vi "test global access to variables.vi"(1 "command":enum16{"read", "write"}(ring), 2 "Current Control settings":T1 {"Pump speed" format="%.2f"}) -> (0 "Current Control settings out":T1 {"Pump speed" format="%.2f"})   [LabVIEW 2010]
uses:
  Stamp Controls.ctl
  switches.ctl
panel:
  # "rpm"
  # "rpm"
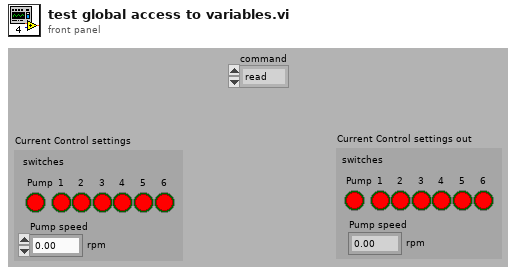
[diagram p1: front panel]
types:
  T1 = typedef "Stamp Controls.ctl" = cluster{"Pump speed":dbl, "switches":T2}
  T2 = typedef "switches.ctl" = cluster{"Pump":bool, "1":bool, "2":bool, "3":bool, "4":bool, "5":bool, "6":bool}
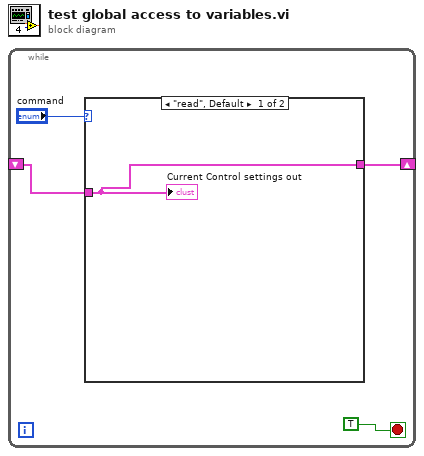
[diagram p0: block diagram]
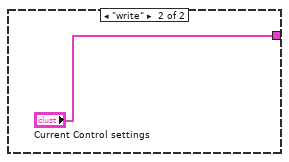
[diagram p2: hidden frame]
diagram:
  n1 = while {
    shift-right: [w3] -> _
    shift-left: _ -> [w2]
    stop <- TRUE stop-if-true
    n2 = case shown="\"read\", Default" "command" {
      tunnel: [w5 "Current Control settings"] -> w3
      tunnel: w2 -> [w5 _]
      frame "read", Default {
        "Current Control settings out" <- w5
      }
      frame "write" {
      }
    }
  }
